vi "Toggle.vi"(11 "NewVal":bool) -> (3 "NewVal2":bool)   [LabVIEW 2014]
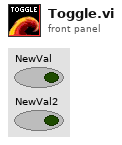
[diagram p1: front panel]
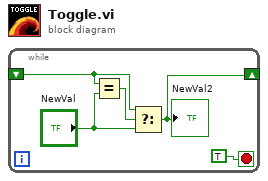
[diagram p0: block diagram]
diagram:
  n1 = while {
    shift-right: [w1] -> _
    shift-left: _ -> [w2]
    stop <- TRUE stop-if-true
    n2 = Equal?(x=w2, y="NewVal") -> (x = y?=w4:bool)
    n3 = Select(t=w2, s=w4, f="NewVal") -> (s? t:f=w1:bool)
    "NewVal2" <- w1
  }
